vi "UpdateTestingResults.vi"(8 "Variant":string, 9 "SerialNumber":string, 10 "NewData":u8[](array[numeric]), 11 "index (row)":i32) -> ()   [LabVIEW 2023]
uses:
  <vilib>/Utility/file.llb/Read Delimited Spreadsheet (I64).vi
  <vilib>/Utility/file.llb/Write Delimited Spreadsheet (I64).vi
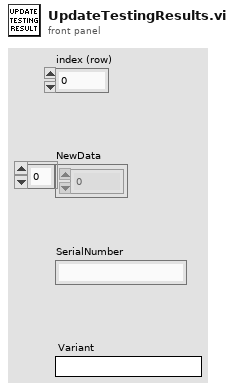
[diagram p1: front panel]
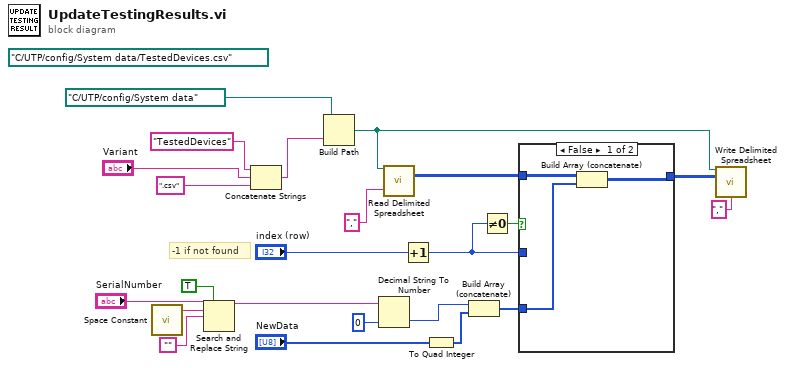
[diagram p0: block diagram]
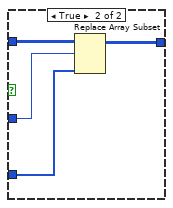
[diagram p2: hidden frame]
diagram:
  (unwired) path "C:/UTP/config/System data/TestedDevices.csv" ("file path (dialog if empty)")
  # "-1 if not found"
  n1 = call <vilib>:"Space Constant.vi"() -> ("String"=w5:string)
  n2 = Search and Replace String(replace all?=TRUE ("replace all? (F)"), input string="SerialNumber", search string=w5, replace string="") -> (result string=w3:string)  [unwired: 4 in, 3 out]
  n3 = Concatenate Strings("TestedDevices" ("string"), "Variant", ".csv" ("string")) -> (w9:string)
  n4 = Build Path(base path=path "C:/UTP/config/System data" ("file path (dialog if empty)"), name or relative path=w9) -> (appended path=w7:path)
  n5 = Decimal String To Number(string=w3, default (0L)=i64 0) -> (number=w18:i64)  [unwired: 1 in, 1 out]
  n6 = call-poly <vilib>:"Read Delimited Spreadsheet.vi"("file path (dialog if empty)"=w7, "delimiter (\\t)"="," ("delimiter (\\t)")) -> ("all rows"=w14:i64[][])  [unwired: 8 in, 5 out]
  n7 = Increment(x="index (row)") -> (x+1=w12:i32)
  n8 = To Quad Integer(1:"NewData") -> (0:w15:i64[])
  n9 = Build Array (concatenate)(w18, w15) -> (w16:i64[])
  n10 = Not Equal To 0?(x=w12) -> (x != 0?=w13:bool)
  n11 = case shown="False" w13 {
    tunnel: [w25 w30] -> w21
    tunnel: w16 -> [w24 w29]
    tunnel: w14 -> [w26 w28]
    tunnel: w12 -> [_ w27]
    frame False {
      n12 = Build Array (concatenate)(w26, w24) -> (w25:i64[][])
    }
    frame True {
      n13 = Replace Array Subset(array=w28, new element=w29, index (row)=w27) -> (w30:i64[][])  [unwired: 1 in]
    }
  }
  n14 = call-poly <vilib>:"Write Delimited Spreadsheet.vi"("file path (dialog if empty)"=w7, "2D data"=w21, "delimiter (\\t)"="," ("delimiter (\\t)")) -> ()  [unwired: 11 in, 2 out]
